vi "credit update.vi"(8 "error in (no error)":errorcluster, 10 "credito":dbl, 11 "UI Actor in":refnum<class "UI Actor.lvclass">) -> (0 "error out":errorcluster, 3 "UI Actor out":refnum<class "UI Actor.lvclass">)   [LabVIEW 2020, in "UI Actor.lvlib" / "UI Actor.lvclass"]
uses:
  UI Actor.lvclass
  UI Actor.lvclass/UI Actor.ctl
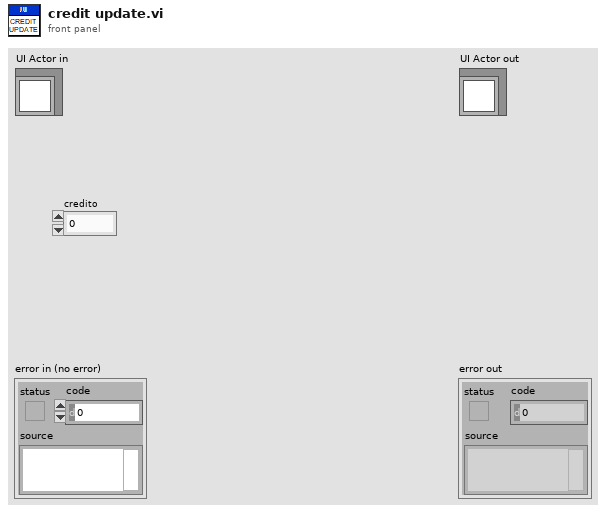
[diagram p1: front panel]
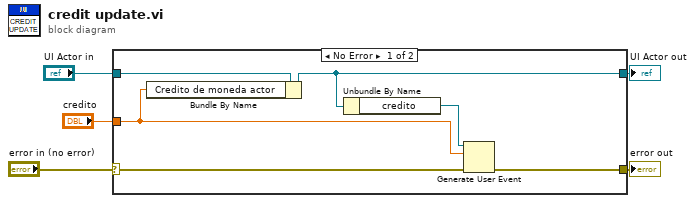
[diagram p0: block diagram]
diagram:
  n1 = case shown="No Error" "error in (no error)" {
    selector: "error in (no error)" -> [w9 w13]
    tunnel: [w8 w13] -> w4
    tunnel: [w7 w12] -> w2
    tunnel: "UI Actor in" -> [w11 w12]
    tunnel: "credito" -> [w6 _]
    frame No Error {
      n2 = Bundle By Name(cluster=w11, "Credito de moneda actor"=w6) -> (w7:refnum<class "UI Actor.lvclass">)
      n3 = Unbundle By Name(w7) -> ("credito"=w10:refnum<user-event>)
      n4 = Generate User Event(user event=w10, event data cluster=w6, error in=w9) -> (error out=w8:errorcluster)  [unwired: 1 in, 1 out]
    }
    frame Error {
    }
  }
  "error out" <- w4
  "UI Actor out" <- w2
